vi "DiffDriveOdom_RelativeTrajectory_ProcessAuto.vi"   [LabVIEW 2019]
uses:
  <vilib>/Rock Robotics/WPI/ThirdParty/JAS_Junk/TrajLib/VI/BoolCmd_Recv_Internal.vi
  <vilib>/Rock Robotics/WPI/ThirdParty/JAS_Junk/TrajLib/VI/BoolCmd_ObtainQueue.vi
  Differential Drive Pose Estimator/SubVI/Trajectory_Execution_Diff_Drive/DiffDrivePoseEst2_RelativeTrajectory_Globals.vi
  <vilib>/Rock Robotics/WPI/ThirdParty/JAS_Junk/TrajLib/Trajectory_Library.lvlib
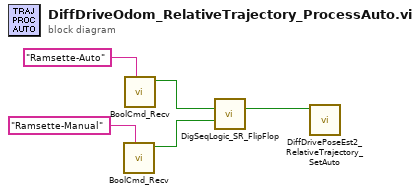
[diagram p0: block diagram]
diagram:
  n1 = call <vilib>:"BoolCmd_Recv.vi"("Command Name"="Ramsette-Manual") -> ("New Request"=w2:bool)  [unwired: 9 in, 1 out]
  n2 = call <vilib>:"BoolCmd_Recv.vi"("Command Name"="Ramsette-Auto") -> ("New Request"=w3:bool)  [unwired: 9 in, 1 out]
  n3 = call <vilib>:"DigSeqLogic_SR_FlipFlop.vi"("Set"=w3, "Reset"=w2) -> ("Output"=w1:bool)  [unwired: 12 in, 1 out]
  n4 = call "DiffDrivePoseEst2_RelativeTrajectory_SetAuto.vi"("Ramsete AUTO"=w1) -> ()  [unwired: 11 in]
